vi "Set Attributes Priv.vi"(0 "Tree Dictionary Out":variant, 5 "Unique ID":string, 7 "Data":variant, 9 "Name":string, 11 "error in":errorcluster) -> (4 "Tree Dictionary Out":variant, 8 "Replaced?":bool, 15 "error out":errorcluster)   [LabVIEW 2016, in "Tree Manager.lvclass"]
uses:
  Tree Manager.lvclass
  Typedefs/Tree.ctl
  <vilib>/Utility/error.llb/Error Cluster From Error Code.vi
  <vilib>/ErrorRing/Error Ring.xnode
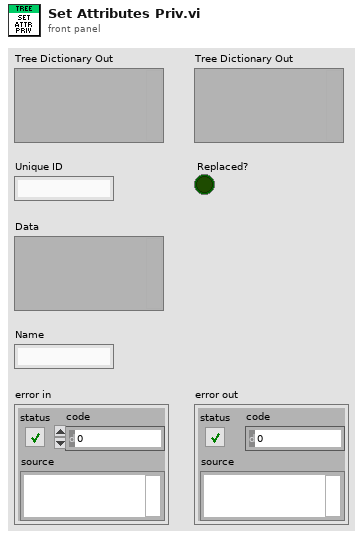
[diagram p1: front panel]
types:
  T1 = typedef "Tree Manager.lvclass/Tree.ctl" = cluster{"Unique ID":string, "Parent ID":string, "Child IDs":string[], "Data":variant, "Name":string}
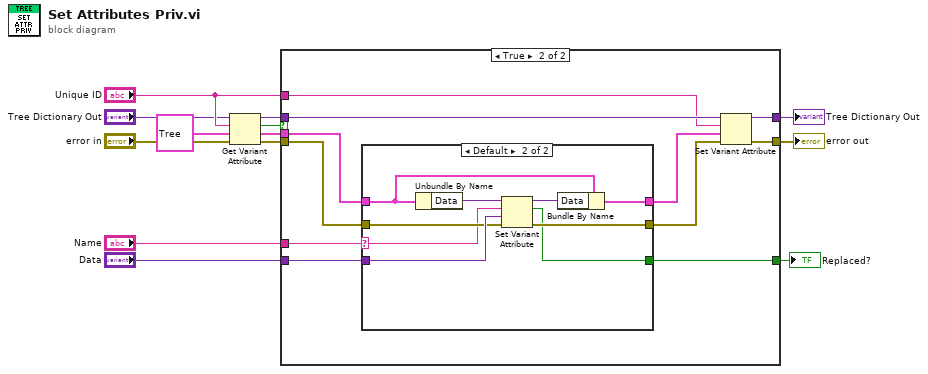
[diagram p0: block diagram]
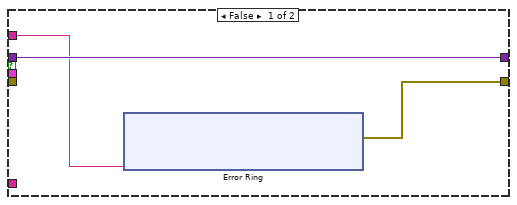
[diagram p2: hidden frame]
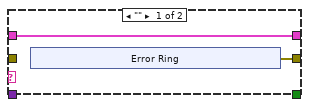
[diagram p3: hidden frame]
diagram:
  n1 = Get Variant Attribute(Variant="Tree Dictionary Out", name="Unique ID", default value (empty Variant)=T1 {"Unique ID"="", "Parent ID"="", "Child IDs"=[], "Data"=variant, "Name"=""} ("Cluster of class private data"), error in="error in") -> (duplicate Variant=w8:variant, found=w9:bool, value=w10:T1, error out=w6:errorcluster)
  n2 = case shown="True" w9 {
    tunnel: [w15 w34] -> w4
    tunnel: [w16 w33] -> w5
    tunnel: w6 -> [_ w30]
    tunnel: w8 -> [w16 w32]
    tunnel: w10 -> [_ w26]
    tunnel: "Name" -> [_ w28]
    tunnel: "Data" -> [_ w31]
    tunnel: "Unique ID" -> [w14 w27]
    tunnel: [_ w24] -> w2
    frame False {
      n3 = xnode "Error Ring"("parameter 0"=w14) -> ("error out"=w15:errorcluster)
    }
    frame True {
      n4 = case shown="Default" w28 {
        selector: w28 -> [_ w46]
        tunnel: w31 -> [_ w49]
        tunnel: w30 -> [_ w48]
        tunnel: [w36 w47] -> w29
        tunnel: w26 -> [w35 w45]
        tunnel: [w35 w43] -> w25
        tunnel: [_ w42] -> w24
        frame "" {
          n5 = xnode "Error Ring"() -> ("error out"=w36:errorcluster)
        }
        frame Default {
          n6 = Unbundle By Name(w45) -> ("Data"=w44:variant)
          n7 = Set Variant Attribute(Variant=w44, name=w46, value=w49, error in=w48) -> (Variant out=w50:variant, replaced=w42:bool, error out=w47:errorcluster)
          n8 = Bundle By Name(cluster=w45, "Data"=w50) -> (w43:T1)
        }
      }
      n9 = Set Variant Attribute(Variant=w32, name=w27, value=w25, error in=w29) -> (Variant out=w33:variant, error out=w34:errorcluster)  [unwired: 1 out]
    }
  }
  "Tree Dictionary Out" <- w5
  "error out" <- w4
  "Replaced?" <- w2
